vi "FMA1600A Dryer Data Build.vi"(7 "Barometric Pressure.Barometric Pressure (in. Hg)":dbl, 8 "Error In":errorcluster, 11 "DAQ Data In in":T1={"Meter 1"={"Meter Size"=0.0, "DAQ Output (Voltage)"=0.0, "Reference (Voltage)"=0.0, "Meter Present"=FALSE, "Meter Visa"="COM3", "Gas Type"="", "SLPM Error @ Zero"=0.0, "Gas Mix Number"="", "Set STP Register"=FALSE, "Measurement Units"={"Software Rev"="", "Model Number"="", "Manufacturer Info"="", "Software Sub-Rev"="", "Board Rev"="", "Units of Measure Input"={"Abs. Pressure"="", "Gauge/Diff. Press."="", "Barometric Press."="", "Temperature"="", "Volume"="", "Mass"="", "Setpoint"="", "Valve Drive"="", "Totalizer"="", "Tot. Timer"="", "Tot. Avg. Flow"="", "Tot. Peak Flow"=""}}, "Data Frame Format"={"Absolute Pressure"=FALSE, "Gauge/Diff. Pressure"=FALSE, "Barometric Pressure"=FALSE, "Temperature"=FALSE, "Volumetric"=FALSE, "Mass"=FALSE, "Setpoint"=FALSE, "Valve Drive"=FALSE, "Totalizer"=FALSE, "Totalizer Timer"=FALSE, "Totalizer Average Flow"=FALSE, "Totalizer Peak Flow"=FALSE, "Gas Selected"=FALSE, "Tot. Timer Format"=0}}, "Meter 2"={"Meter Size"=0.0, "DAQ Output (Voltage)"=0.0, "Reference (Voltage)"=0.0, "Meter Present"=FALSE, "Meter Visa"="COM3", "Gas Type"="", "SLPM Error @ Zero"=0.0, "Gas Mix Number"="", "Set STP Register"=FALSE, "Measurement Units"={"Software Rev"="", "Model Number"="", "Manufacturer Info"="", "Software Sub-Rev"="", "Board Rev"="", "Units of Measure Input"={"Abs. Pressure"="", "Gauge/Diff. Press."="", "Barometric Press."="", "Temperature"="", "Volume"="", "Mass"="", "Setpoint"="", "Valve Drive"="", "Totalizer"="", "Tot. Timer"="", "Tot. Avg. Flow"="", "Tot. Peak Flow"=""}}, "Data Frame Format"={"Absolute Pressure"=FALSE, "Gauge/Diff. Pressure"=FALSE, "Barometric Pressure"=FALSE, "Temperature"=FALSE, "Volumetric"=FALSE, "Mass"=FALSE, "Setpoint"=FALSE, "Valve Drive"=FALSE, "Totalizer"=FALSE, "Totalizer Timer"=FALSE, "Totalizer Average Flow"=FALSE, "Totalizer Peak Flow"=FALSE, "Gas Selected"=FALSE, "Tot. Timer Format"=0}}, "Meter 3"={"Meter Size"=0.0, "DAQ Output (Voltage)"=0.0, "Reference (Voltage)"=0.0, "Meter Present"=FALSE, "Meter Visa"="COM3", "Gas Type"="", "SLPM Error @ Zero"=0.0, "Gas Mix Number"="", "Set STP Register"=FALSE, "Measurement Units"={"Software Rev"="", "Model Number"="", "Manufacturer Info"="", "Software Sub-Rev"="", "Board Rev"="", "Units of Measure Input"={"Abs. Pressure"="", "Gauge/Diff. Press."="", "Barometric Press."="", "Temperature"="", "Volume"="", "Mass"="", "Setpoint"="", "Valve Drive"="", "Totalizer"="", "Tot. Timer"="", "Tot. Avg. Flow"="", "Tot. Peak Flow"=""}}, "Data Frame Format"={"Absolute Pressure"=FALSE, "Gauge/Diff. Pressure"=FALSE, "Barometric Pressure"=FALSE, "Temperature"=FALSE, "Volumetric"=FALSE, "Mass"=FALSE, "Setpoint"=FALSE, "Valve Drive"=FALSE, "Totalizer"=FALSE, "Totalizer Timer"=FALSE, "Totalizer Average Flow"=FALSE, "Totalizer Peak Flow"=FALSE, "Gas Selected"=FALSE, "Tot. Timer Format"=0}}, "Meter 4"={"Meter Size"=0.0, "DAQ Output (Voltage)"=0.0, "Reference (Voltage)"=0.0, "Meter Present"=FALSE, "Meter Visa"="COM3", "Gas Type"="", "SLPM Error @ Zero"=0.0, "Gas Mix Number"="", "Set STP Register"=FALSE, "Measurement Units"={"Software Rev"="", "Model Number"="", "Manufacturer Info"="", "Software Sub-Rev"="", "Board Rev"="", "Units of Measure Input"={"Abs. Pressure"="", "Gauge/Diff. Press."="", "Barometric Press."="", "Temperature"="", "Volume"="", "Mass"="", "Setpoint"="", "Valve Drive"="", "Totalizer"="", "Tot. Timer"="", "Tot. Avg. Flow"="", "Tot. Peak Flow"=""}}, "Data Frame Format"={"Absolute Pressure"=FALSE, "Gauge/Diff. Pressure"=FALSE, "Barometric Pressure"=FALSE, "Temperature"=FALSE, "Volumetric"=FALSE, "Mass"=FALSE, "Setpoint"=FALSE, "Valve Drive"=FALSE, "Totalizer"=FALSE, "Totalizer Timer"=FALSE, "Totalizer Average Flow"=FALSE, "Totalizer Peak Flow"=FALSE, "Gas Selected"=FALSE, "Tot. Timer Format"=0}}, "Meter 5"={"Meter Size"=0.0, "DAQ Output (Voltage)"=0.0, "Reference (Voltage)"=0.0, "Meter Present"=FALSE, "Meter Visa"="COM3", "Gas Type"="", "SLPM Error @ Zero"=0.0, "Gas Mix Number"="", "Set STP Register"=FALSE, "Measurement Units"={"Software Rev"="", "Model Number"="", "Manufacturer Info"="", "Software Sub-Rev"="", "Board Rev"="", "Units of Measure Input"={"Abs. Pressure"="", "Gauge/Diff. Press."="", "Barometric Press."="", "Temperature"="", "Volume"="", "Mass"="", "Setpoint"="", "Valve Drive"="", "Totalizer"="", "Tot. Timer"="", "Tot. Avg. Flow"="", "Tot. Peak Flow"=""}}, "Data Frame Format"={"Absolute Pressure"=FALSE, "Gauge/Diff. Pressure"=FALSE, "Barometric Pressure"=FALSE, "Temperature"=FALSE, "Volumetric"=FALSE, "Mass"=FALSE, "Setpoint"=FALSE, "Valve Drive"=FALSE, "Totalizer"=FALSE, "Totalizer Timer"=FALSE, "Totalizer Average Flow"=FALSE, "Totalizer Peak Flow"=FALSE, "Gas Selected"=FALSE, "Tot. Timer Format"=0}}, "Meter 6"={"Meter Size"=0.0, "DAQ Output (Voltage)"=0.0, "Reference (Voltage)"=0.0, "Meter Present"=FALSE, "Meter Visa"="COM3", "Gas Type"="", "SLPM Error @ Zero"=0.0, "Gas Mix Number"="", "Set STP Register"=FALSE, "Measurement Units"={"Software Rev"="", "Model Number"="", "Manufacturer Info"="", "Software Sub-Rev"="", "Board Rev"="", "Units of Measure Input"={"Abs. Pressure"="", "Gauge/Diff. Press."="", "Barometric Press."="", "Temperature"="", "Volume"="", "Mass"="", "Setpoint"="", "Valve Drive"="", "Totalizer"="", "Tot. Timer"="", "Tot. Avg. Flow"="", "Tot. Peak Flow"=""}}, "Data Frame Format"={"Absolute Pressure"=FALSE, "Gauge/Diff. Pressure"=FALSE, "Barometric Pressure"=FALSE, "Temperature"=FALSE, "Volumetric"=FALSE, "Mass"=FALSE, "Setpoint"=FALSE, "Valve Drive"=FALSE, "Totalizer"=FALSE, "Totalizer Timer"=FALSE, "Totalizer Average Flow"=FALSE, "Totalizer Peak Flow"=FALSE, "Gas Selected"=FALSE, "Tot. Timer Format"=0}}, "Meter Bank 1"={"Flow Rate (BTU/HR)"=0.0, "ANSI Average (BTU/HR)"=0.0, "Panel Data"={"Meter Type (Gas)"="", "Heating Value (BTU/ft³)"=0.0, "Ft³ / Hr (SCFH)"=0.0, "15 Second Average (BTU/HR)"=0.0, "30 Second Average (BTU/HR)"=0.0, "Mass Flow"=0.0, "Vol. Flow"=0.0, "Gas Temperature"=0.0, "Gas Pressure"=0.0, "Tot.Flow"=0.0}, "Meter ID"="", "ANSI Rate"={"Array 1"=[], "Array 3"=[], "Array 2"=[], "Start ANSI"=FALSE, "ANSI Start Time"=0.0, "Restart ANSI"=FALSE, "15 Min ANSI Avg (BTU/hr)"=0.0, "20 Min ANSI Avg (BTU/hr)"=0.0, "25 Min ANSI Avg (BTU/hr)"=0.0, "Absolute Pressure"=0.0, "Gas Temperature"=0.0, "Volumetric Flow Rate"=0.0, "Mass Flow Rate"=0.0, "Array 4"=[], "Array 5"=[], "Gas Rate"=0.0, "15 Min Pres Avg (PSIA)"=0.0, "20 Min Pres Avg (PSIA)"=0.0, "25 Min Pres Avg (PSIA)"=0.0, "15 Min Temp Avg (°F) "=0.0, "20 Min Temp Avg (°F)"=0.0, "25 Min Temp Avg (°F)"=0.0, "15 Min Uncorrected Avg (CFH)"=0.0, "20 Min Uncorrected Avg (CFH)"=0.0, "25 Min Uncorrected Avg (CFH)"=0.0, "15 Min Corrected Avg (SCFH)"=0.0, "20 Min Corrected Avg (SCFH)"=0.0, "25 Min Corrected Avg (SCFH)"=0.0, "15 Min Complete"=FALSE, "20 Min Complete"=FALSE, "25 Min Complete"=FALSE, "Heating Value (BTU/ft³)"=0.0, "CO CO2 15 Min"=[], "CO CO2 20 Min"=[], "CO CO2 25 Min"=[], "CO CO2 Real Time"=[]}}, "Meter Bank 2"={"Flow Rate (BTU/HR)"=0.0, "ANSI Average (BTU/HR)"=0.0, "Panel Data"={"Meter Type (Gas)"="", "Heating Value (BTU/ft³)"=0.0, "Ft³ / Hr (SCFH)"=0.0, "15 Second Average (BTU/HR)"=0.0, "30 Second Average (BTU/HR)"=0.0, "Mass Flow"=0.0, "Vol. Flow"=0.0, "Gas Temperature"=0.0, "Gas Pressure"=0.0, "Tot.Flow"=0.0}, "Meter ID"="", "ANSI Rate"={"Array 1"=[], "Array 3"=[], "Array 2"=[], "Start ANSI"=FALSE, "ANSI Start Time"=0.0, "Restart ANSI"=FALSE, "15 Min ANSI Avg (BTU/hr)"=0.0, "20 Min ANSI Avg (BTU/hr)"=0.0, "25 Min ANSI Avg (BTU/hr)"=0.0, "Absolute Pressure"=0.0, "Gas Temperature"=0.0, "Volumetric Flow Rate"=0.0, "Mass Flow Rate"=0.0, "Array 4"=[], "Array 5"=[], "Gas Rate"=0.0, "15 Min Pres Avg (PSIA)"=0.0, "20 Min Pres Avg (PSIA)"=0.0, "25 Min Pres Avg (PSIA)"=0.0, "15 Min Temp Avg (°F) "=0.0, "20 Min Temp Avg (°F)"=0.0, "25 Min Temp Avg (°F)"=0.0, "15 Min Uncorrected Avg (CFH)"=0.0, "20 Min Uncorrected Avg (CFH)"=0.0, "25 Min Uncorrected Avg (CFH)"=0.0, "15 Min Corrected Avg (SCFH)"=0.0, "20 Min Corrected Avg (SCFH)"=0.0, "25 Min Corrected Avg (SCFH)"=0.0, "15 Min Complete"=FALSE, "20 Min Complete"=FALSE, "25 Min Complete"=FALSE, "Heating Value (BTU/ft³)"=0.0, "CO CO2 15 Min"=[], "CO CO2 20 Min"=[], "CO CO2 25 Min"=[], "CO CO2 Real Time"=[]}}, "Meter Bank 3"={"Flow Rate (BTU/HR)"=0.0, "ANSI Average (BTU/HR)"=0.0, "Panel Data"={"Meter Type (Gas)"="", "Heating Value (BTU/ft³)"=0.0, "Ft³ / Hr (SCFH)"=0.0, "15 Second Average (BTU/HR)"=0.0, "30 Second Average (BTU/HR)"=0.0, "Mass Flow"=0.0, "Vol. Flow"=0.0, "Gas Temperature"=0.0, "Gas Pressure"=0.0, "Tot.Flow"=0.0}, "Meter ID"="", "ANSI Rate"={"Array 1"=[], "Array 3"=[], "Array 2"=[], "Start ANSI"=FALSE, "ANSI Start Time"=0.0, "Restart ANSI"=FALSE, "15 Min ANSI Avg (BTU/hr)"=0.0, "20 Min ANSI Avg (BTU/hr)"=0.0, "25 Min ANSI Avg (BTU/hr)"=0.0, "Absolute Pressure"=0.0, "Gas Temperature"=0.0, "Volumetric Flow Rate"=0.0, "Mass Flow Rate"=0.0, "Array 4"=[], "Array 5"=[], "Gas Rate"=0.0, "15 Min Pres Avg (PSIA)"=0.0, "20 Min Pres Avg (PSIA)"=0.0, "25 Min Pres Avg (PSIA)"=0.0, "15 Min Temp Avg (°F) "=0.0, "20 Min Temp Avg (°F)"=0.0, "25 Min Temp Avg (°F)"=0.0, "15 Min Uncorrected Avg (CFH)"=0.0, "20 Min Uncorrected Avg (CFH)"=0.0, "25 Min Uncorrected Avg (CFH)"=0.0, "15 Min Corrected Avg (SCFH)"=0.0, "20 Min Corrected Avg (SCFH)"=0.0, "25 Min Corrected Avg (SCFH)"=0.0, "15 Min Complete"=FALSE, "20 Min Complete"=FALSE, "25 Min Complete"=FALSE, "Heating Value (BTU/ft³)"=0.0, "CO CO2 15 Min"=[], "CO CO2 20 Min"=[], "CO CO2 25 Min"=[], "CO CO2 Real Time"=[]}}, "Threshold Voltage (NI DAQ)"=0.0, "Use RS232 Data Collection"=FALSE, "Use Auto Switching"=FALSE}) -> (0 "Error Out":errorcluster, 2 "LPM (Vol. Flow)":dbl, 3 "Dryer Data":string[][](array[string]))   [LabVIEW 2019]
uses:
  Trunk/Range/Type Definitions/RANGE DAQ Data Four Meters.ctl
  Trunk/Range/Type Definitions/RANGE DAQ Data.ctl
  Type Definitions/FMA1600A Gas Type.ctl
  Type Definitions/FMA1600A Units String.ctl
  Alicat Gas Meter Driver/Sub-VIs/Units of Measure.ctl
  Alicat Gas Meter Driver/Sub-VIs/Data Frame.ctl
  Trunk/Range/Type Definitions/RANGE GAS Data.ctl
  Trunk/Range/Type Definitions/RANGE Panel Data.ctl
  Trunk/Range/Type Definitions/RANGE ANSI Rate.ctl
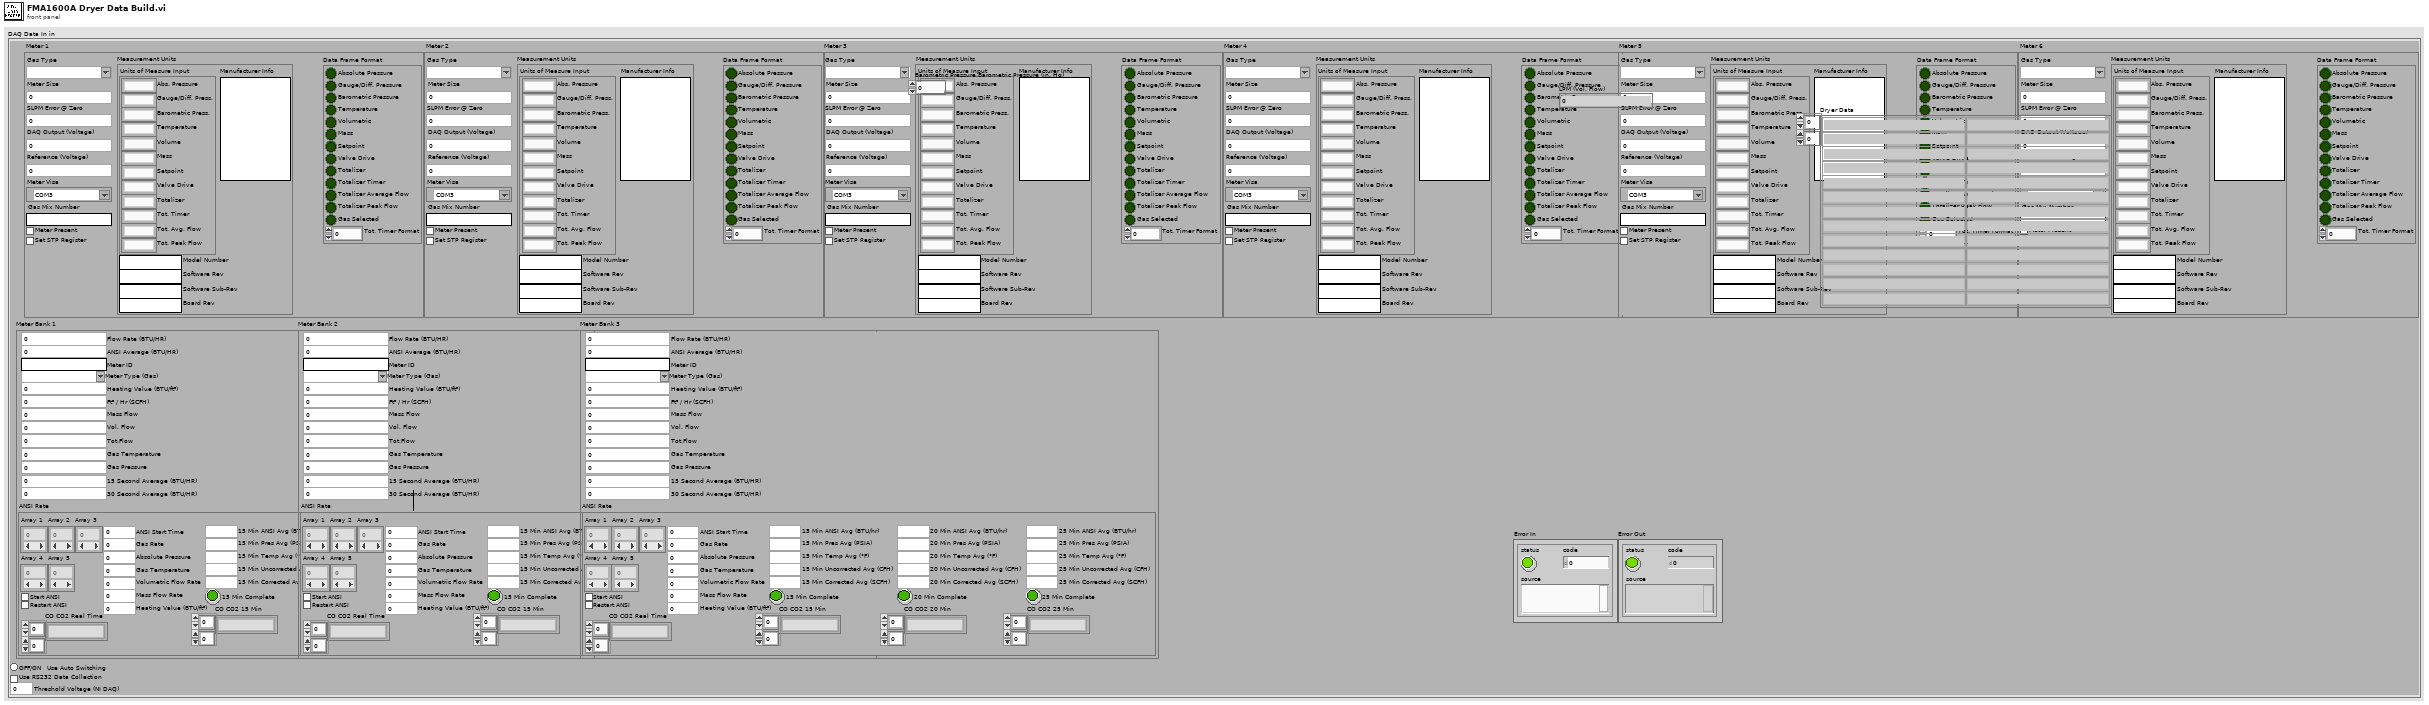
[diagram p1: front panel]
types:
  T1 = typedef "RANGE DAQ Data Four Meters.ctl" = cluster{"Meter 1":T2, "Meter 2":T2, "Meter 3":T2, "Meter 4":T2, "Meter 5":T2, "Meter 6":T2, "Meter Bank 1":T7, "Meter Bank 2":T7, "Meter Bank 3":T7, "Threshold Voltage (NI DAQ)":dbl, "Use RS232 Data Collection":bool, "Use Auto Switching":bool}
  T2 = typedef "RANGE DAQ Data.ctl" = cluster{"Meter Size":dbl, "DAQ Output (Voltage)":dbl, "Reference (Voltage)":dbl, "Meter Present":bool, "Meter Visa":refnum<visa-resource-name>, "Gas Type":T3, "SLPM Error @ Zero":dbl, "Gas Mix Number":string, "Set STP Register":bool, "Measurement Units":T4, "Data Frame Format":T6}
  T3 = typedef "FMA1600A Gas Type.ctl" = string
  T4 = typedef "FMA1600A Units String.ctl" = cluster{"Software Rev":string, "Model Number":string, "Manufacturer Info":string, "Software Sub-Rev":string, "Board Rev":string, "Units of Measure Input":T5}
  T5 = typedef "Units of Measure.ctl" = cluster{"Abs. Pressure":string, "Gauge/Diff. Press.":string, "Barometric Press.":string, "Temperature":string, "Volume":string, "Mass":string, "Setpoint":string, "Valve Drive":string, "Totalizer":string, "Tot. Timer":string, "Tot. Avg. Flow":string, "Tot. Peak Flow":string}
  T6 = typedef "Data Frame.ctl" = cluster{"Absolute Pressure":bool, "Gauge/Diff. Pressure":bool, "Barometric Pressure":bool, "Temperature":bool, "Volumetric":bool, "Mass":bool, "Setpoint":bool, "Valve Drive":bool, "Totalizer":bool, "Totalizer Timer":bool, "Totalizer Average Flow":bool, "Totalizer Peak Flow":bool, "Gas Selected":bool, "Tot. Timer Format":u16}
  T7 = typedef "RANGE GAS Data.ctl" = cluster{"Flow Rate (BTU/HR)":dbl, "ANSI Average (BTU/HR)":dbl, "Panel Data":T8, "Meter ID":string, "ANSI Rate":T9}
  T8 = typedef "RANGE Panel Data.ctl" = cluster{"Meter Type (Gas)":T3, "Heating Value (BTU/ft³)":dbl, "Ft³ / Hr (SCFH)":dbl, "15 Second Average (BTU/HR)":dbl, "30 Second Average (BTU/HR)":dbl, "Mass Flow":dbl, "Vol. Flow":dbl, "Gas Temperature":dbl, "Gas Pressure":dbl, "Tot.Flow":dbl}
  T9 = typedef "RANGE ANSI Rate.ctl" = cluster{"Array 1":dbl[], "Array 3":dbl[], "Array 2":dbl[], "Start ANSI":bool, "ANSI Start Time":dbl, "Restart ANSI":bool, "15 Min ANSI Avg (BTU/hr)":dbl, "20 Min ANSI Avg (BTU/hr)":dbl, "25 Min ANSI Avg (BTU/hr)":dbl, "Absolute Pressure":dbl, "Gas Temperature":dbl, "Volumetric Flow Rate":dbl, "Mass Flow Rate":dbl, "Array 4":dbl[], "Array 5":dbl[], "Gas Rate":dbl, "15 Min Pres Avg (PSIA)":dbl, "20 Min Pres Avg (PSIA)":dbl, "25 Min Pres Avg (PSIA)":dbl, "15 Min Temp Avg (°F) ":dbl, "20 Min Temp Avg (°F)":dbl, "25 Min Temp Avg (°F)":dbl, "15 Min Uncorrected Avg (CFH)":dbl, "20 Min Uncorrected Avg (CFH)":dbl, "25 Min Uncorrected Avg (CFH)":dbl, "15 Min Corrected Avg (SCFH)":dbl, "20 Min Corrected Avg (SCFH)":dbl, "25 Min Corrected Avg (SCFH)":dbl, "15 Min Complete":bool, "20 Min Complete":bool, "25 Min Complete":bool, "Heating Value (BTU/ft³)":dbl, "CO CO2 15 Min":string[][], "CO CO2 20 Min":string[][], "CO CO2 25 Min":string[][], "CO CO2 Real Time":string[][]}
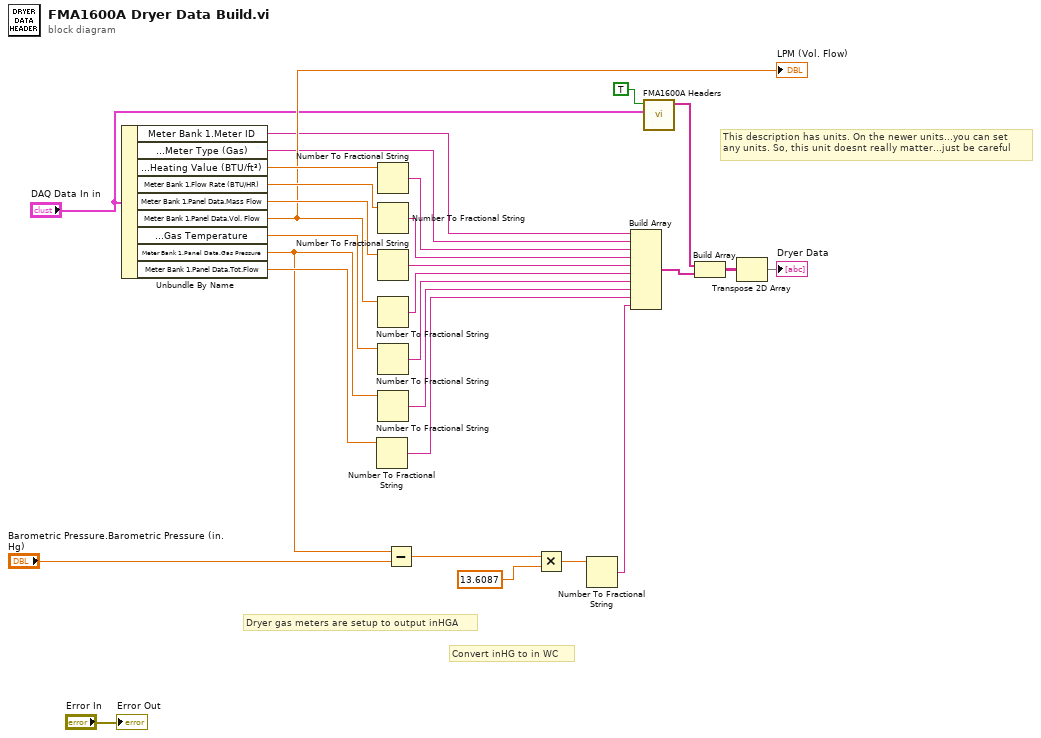
[diagram p0: block diagram]
diagram:
  # "This description has units. On the newer units...you can set\nany units. So, this unit doesnt really matter...just be careful"
  # "Convert inHG to in WC"
  # "Dryer gas meters are setup to output inHGA"
  n1 = Unbundle By Name("DAQ Data In in") -> ("Meter Bank 1.Meter ID"=w1:string, "Meter Bank 1.Panel Data.Meter Type (Gas)"=w3:T3, "Meter Bank 1.Panel Data.Heating Value (BTU/ft³)"=w28:dbl, "Meter Bank 1.Flow Rate (BTU/HR)"=w27:dbl, "Meter Bank 1.Panel Data.Mass Flow"=w26:dbl, "Meter Bank 1.Panel Data.Vol. Flow"=w25:dbl, "Meter Bank 1.Panel Data.Gas Temperature"=w24:dbl, "Meter Bank 1.Panel Data.Gas Pressure"=w9:dbl, "Meter Bank 1.Panel Data.Tot.Flow"=w23:dbl)
  "LPM (Vol. Flow)" <- w25
  n2 = Number To Fractional String(number=w23) -> (F-format string=w16:string)  [unwired: 3 in]
  n3 = Number To Fractional String(number=w28) -> (F-format string=w22:string)  [unwired: 3 in]
  n4 = Number To Fractional String(number=w27) -> (F-format string=w21:string)  [unwired: 3 in]
  n5 = Number To Fractional String(number=w26) -> (F-format string=w20:string)  [unwired: 3 in]
  n6 = Number To Fractional String(number=w25) -> (F-format string=w19:string)  [unwired: 3 in]
  n7 = Number To Fractional String(number=w24) -> (F-format string=w18:string)  [unwired: 3 in]
  n8 = Number To Fractional String(number=w9) -> (F-format string=w17:string)  [unwired: 3 in]
  n9 = Subtract(x=w9, y="Barometric Pressure.Barometric Pressure (in. Hg)") -> (x-y=w7:dbl)
  n10 = Multiply(x=w7, y=13.6087) -> (x*y=w5:dbl)
  n11 = Number To Fractional String(number=w5) -> (F-format string=w4:string)  [unwired: 3 in]
  n12 = Build Array(w1, w3, w22, w21, w20, w19, w18, w17, w16, w4) -> (w15:T3[])
  n13 = call "FMA1600A Headers.vi"("All Meter Data"="DAQ Data In in", "Dryer?"=TRUE) -> ("Range/Dryer Headers 1"=w14:string[])  [unwired: 6 in, 3 out]
  n14 = Build Array(w14, w15) -> (w12:T3[][])
  n15 = Transpose 2D Array(2D array=w12) -> (transposed array=→"Dryer Data":T3[][])
  "Error Out" <- "Error In"
